vi "Um.vi"(0 "x_d":T1, 1 "phi_d":T1, 2 "theta":T1, 3 "error in (no error)":errorcluster, 4 "N":i32) -> (5 "Um":dbl, 6 "error out":errorcluster)   [LabVIEW 2021]
uses:
  <vilib>/Analysis/Matrix/Datatypes/RealMatrix.ctl
  <vilib>/Analysis/Matrix/Numeric/Multiply/Multiply - RM,RM.vi
  <vilib>/Analysis/Matrix/NI_Matrix.lvlib
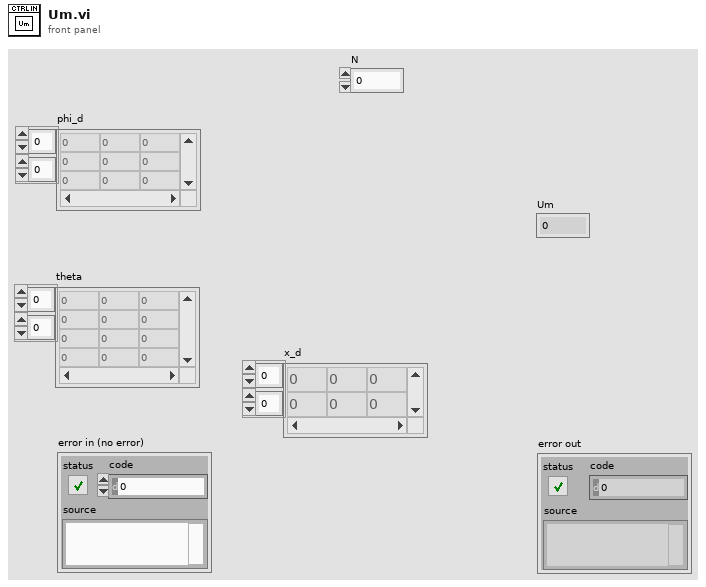
[diagram p1: front panel]
types:
  T1 = typedef "NI_Matrix.lvlib/RealMatrix.ctl" = dbl[][]
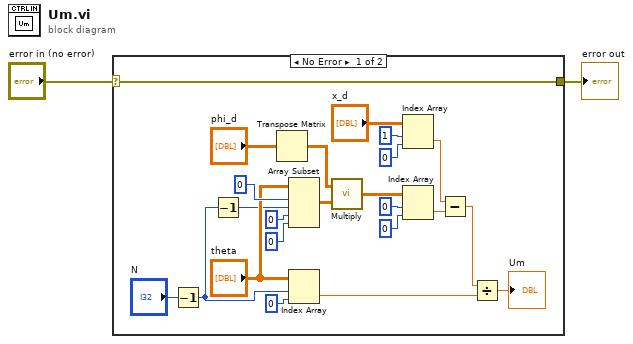
[diagram p0: block diagram]
diagram:
  n1 = case shown="No Error" "error in (no error)" {
    selector: "error in (no error)" -> [w5 w26]
    tunnel: [w5 w26] -> w1
    frame No Error {
      n2 = Decrement(x="N") -> (x-1=w4:i32)
      n3 = Decrement(x=w4) -> (x-1=w3:i32)
      n4 = Transpose Matrix(1:"phi_d") -> (0:w16:T1)
      n5 = Array Subset(array="theta", index (row)=0 ("row 1"), length (row)=w3, index (col)=0 ("column 1"), length (col)=0 ("column N")) -> (w17:T1)
      n6 = Index Array(array="theta", index (row)=w4, index (col)=0) -> (element=w7:dbl)
      n7 = call-poly <vilib>:"Multiply.vi"("Real Matrix B"=w17, "Real Matrix A"=w16) -> ("A * B"=w15:T1)
      n8 = Index Array(array="x_d", index (row)=1, index (col)=0) -> (element=w22:dbl)
      n9 = Index Array(array=w15, index (row)=0, index (col)=0) -> (element=w12:dbl)
      n10 = Subtract ("Subtract.vi")(x=w22, y=w12) -> (x-y=w8:dbl)
      n11 = Divide(x=w8, y=w7) -> (x/y=→"Um":dbl)
    }
    frame Error {
    }
  }
  "error out" <- w1
